vi "Add Stock Price.vi"(9 "Trends":dbl[](array[numeric]), 10 "Fluctuation":dbl, 11 "Stocks Prices":dbl[][](array[numeric])) -> (3 "Stock Prices out":dbl[][](array[numeric]))   [LabVIEW 2025, in "Full Featured MCP Server.lvlib"]
uses:
  Full Featured MCP Server.lvlib
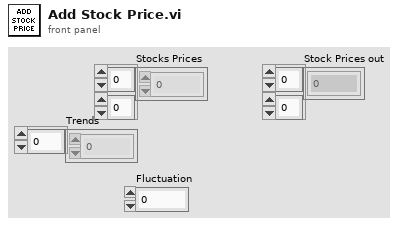
[diagram p1: front panel]
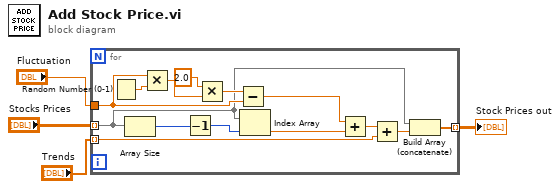
[diagram p0: block diagram]
diagram:
  n1 = for {
    tunnel: "Stocks Prices" -> [w10] mode=indexing
    tunnel: "Fluctuation" -> [w14]
    tunnel: [w9] -> w4 mode=indexing
    tunnel: "Trends" -> [w7] mode=indexing
    n2 = Random Number (0-1)() -> (number: 0 to 1=w18:dbl)
    n3 = Array Size(array=w10) -> (size(s)=w13:i32)
    n4 = Multiply(x=w14, y=w18) -> (x*y=w17:dbl)
    n5 = Decrement(x=w13) -> (x-1=w12:i32)
    n6 = Multiply(x=2.0, y=w17) -> (x*y=w15:dbl)
    n7 = Subtract(x=w15, y=w14) -> (x-y=w5:dbl)
    n8 = Index Array(array=w10, index=w12) -> (element=w11:dbl)
    n9 = Add(x=w5, y=w11) -> (x+y=w6:dbl)
    n10 = Add(x=w6, y=w7) -> (x+y=w8:dbl)
    n11 = Build Array (concatenate)(w10, w8) -> (w9:dbl[])
  }
  "Stock Prices out" <- w4
